vi "tc.vi"(7 "input":dbl, 8 "Tau":dbl=9.49, 10 "Kss":dbl=1.1, 11 "T0":dbl) -> (2 "output":dbl)   [LabVIEW 2018]
panel:
  # "This takes the first given input as the \nambient tempeerature."
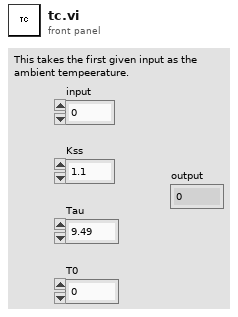
[diagram p1: front panel]
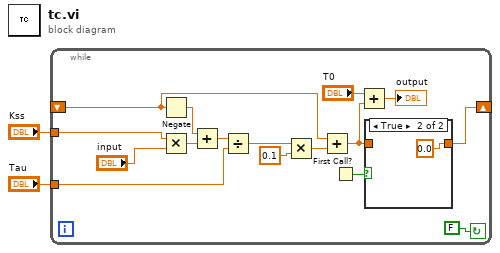
[diagram p0: block diagram]
diagram:
  n1 = while {
    shift-right: [w7] -> _
    shift-left: _ -> [w9]
    tunnel: "Kss" -> [w17]
    tunnel: "Tau" -> [w13]
    stop <- FALSE continue-if-true
    n2 = Negate(x=w9) -> (-x=w16:dbl)
    n3 = Multiply(x=w17, y="input") -> (x*y=w15:dbl)
    n4 = Add(x=w16, y=w15) -> (x+y=w14:dbl)
    n5 = Divide(x=w14, y=w13) -> (x/y=w12:dbl)
    n6 = Multiply(x=w12, y=0.1) -> (x*y=w10:dbl)
    n7 = Add(x=w9, y=w10) -> (x+y=w4:dbl)
    n8 = First Call?() -> (First Call?: T/F=w8:bool)
    n9 = Add(x="T0", y=w4) -> (x+y=→"output":dbl)
    n10 = case shown="True" w8 {
      tunnel: [w19 0.0] -> w7
      tunnel: w4 -> [w19 _]
      frame False {
      }
      frame True {
      }
    }
  }
